vi "read.vi"(8 "error in (no error)":errorcluster, 10 "timeout (ms)":i32=500, 11 "EMTestCWS500N in":refnum<class "EMTestCWS500N.lvclass">) -> (0 "error out":errorcluster, 2 "Return String":string, 3 "EMTestCWS500N out":refnum<class "EMTestCWS500N.lvclass">)   [LabVIEW 2013, in "EMTestCWS500N.lvclass"]
uses:
  EMTestCWS500N.lvclass
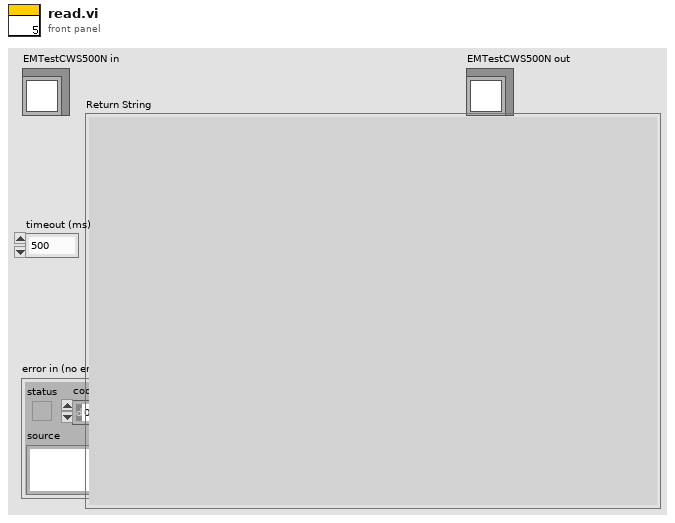
[diagram p1: front panel]
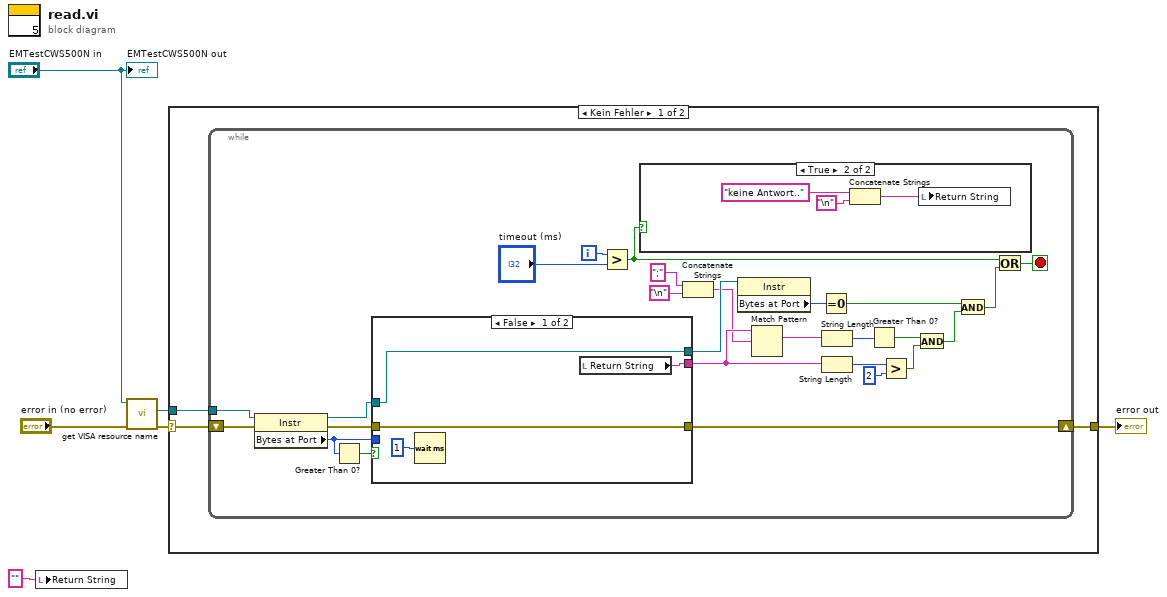
[diagram p0: block diagram]
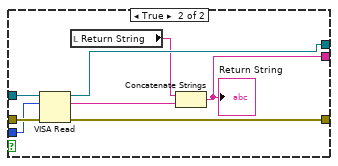
[diagram p3: hidden frame]
diagram:
  n1 = local write "Return String"("") -> ()
  n2 = call-dynamic "get VISA resource name.vi"("error in (no error)"="error in (no error)", "DeviceInterface (Eingang)"="EMTestCWS500N in") -> ("error out"=w1:errorcluster, "VISA resource name"=w3:refnum<visa-resource-name>)  [unwired: 7 in, 1 out]
  n3 = case shown="Kein Fehler" w1 {
    selector: w1 -> [w7 w51]
    tunnel: [w9 w51] -> w6
    tunnel: w3 -> [w8 _]
    frame No Error {
      n4 = while {
        shift-right: [w27] -> w9
        shift-left: w7 -> [w33]
        tunnel: w8 -> [w13]
        i -> [w31]
        stop <- w29 stop-if-true
        n5 = property class="Instr"(reference=w13, error in=w33) -> (reference out=w35:refnum<visa-resource-name>, error out=w34:errorcluster, "Bytes at Port"=w32:u32)
        n6 = Greater Than 0?(x=w32) -> (x > 0?=w30:bool)
        n7 = case shown="False" w30 {
          tunnel: [w41 w50] -> w27
          tunnel: [w42 w49] -> w20
          tunnel: w35 -> [w42 w48]
          tunnel: w34 -> [w41 w47]
          tunnel: w32 -> [_ w44]
          tunnel: [w39 w43] -> w26
          frame False {
            n8 = Wait (ms)(milliseconds to wait=u32 1) -> ()  [unwired: 1 out]
            n9 = local read "Return String"() -> (w39:string)
          }
          frame True {
            n10 = VISA Read(VISA resource name=w48, byte count=w44, error in (no error)=w47) -> (VISA resource name out=w49:refnum<visa-resource-name>, read buffer=w46:string, error out=w50:errorcluster)  [unwired: 1 out]
            n11 = local read "Return String"() -> (w45:string)
            n12 = Concatenate Strings(w45, w46) -> (w43:string)
            "Return String" <- w43
          }
        }
        n13 = Greater?(x=w31, y="timeout (ms)") -> (0:w11:bool)
        n14 = case shown="True" w11 {
          frame False {
          }
          frame True {
            n15 = Concatenate Strings("keine Antwort.." ("Return String"), "\n") -> (w36:string)
            n16 = local write "Return String"(w36) -> ()
          }
        }
        n17 = Concatenate Strings(";" ("regular expression"), "\n") -> (w14:string)
        n18 = property class="Instr"(reference=w20) -> ("Bytes at Port"=w18:u32)  [unwired: 1 in, 2 out]
        n19 = Match Pattern(string=w26, regular expression=w14) -> (match substring=w28:string)  [unwired: 1 in, 3 out]
        n20 = Equal To 0?(x=w18) -> (x = 0?=w19:bool)
        n21 = String Length(string=w28) -> (length=w23:i32)
        n22 = String Length(string=w26) -> (length=w25:i32)
        n23 = Greater Than 0?(x=w23) -> (x > 0?=w22:bool)
        n24 = Greater?(x=w25, y=2) -> (0:w21:bool)
        n25 = And(x=w22, y=w21) -> (x .and. y?=w17:bool)
        n26 = And(x=w19, y=w17) -> (x .and. y?=w10:bool)
        n27 = Or(x=w11, y=w10) -> (x .or. y?=w29:bool)
      }
    }
    frame Error {
    }
  }
  "error out" <- w6
  "EMTestCWS500N out" <- "EMTestCWS500N in"
